vi "xyz-localisation.vi"(5 "Gy":dbl[][](array[numeric]), 7 "Gx":dbl[][](array[numeric]), 8 "R":dbl, 9 "weights":dbl[](array[numeric]), 10 "B points":dbl[][](array[numeric])=[[5.0, 3.0], [6.0, 6.0]], 11 "A points":dbl[][](array[numeric])=[[0.0, 1.0], [2.0, 3.0]]) -> (2 "dR":dbl[](array[numeric]), 3 "XYZ":dbl[](array[numeric]))   [LabVIEW 2015]
doc: "This vi calculates XYZ position of the particle. XY is found as a least square intersection point of gradient lines. Z position is a difference between sum of gradients to the left/bottom and rigth/up sides of particle center (requires calibration)\n\nINPUT\nR - radius of the window (should be >0.5)\nGx,Gy - horizontal and vertical local gradient images\nA points - 2xN array of first points that define lines\nB points - 2xN array of second points that define lines\nw - weights (1D array)\n\nOUTPUT\nXYZ - x,y position of the particle in pixels (for original image), z-value\ndR - distance from the center to each line (1D vector)\n\nAuthor: Anatolii Kashchuk"
panel:
  # "This vi finds centroid and z-value from the image of a particle\n\nAuthor: Anatolii Kashchuk"
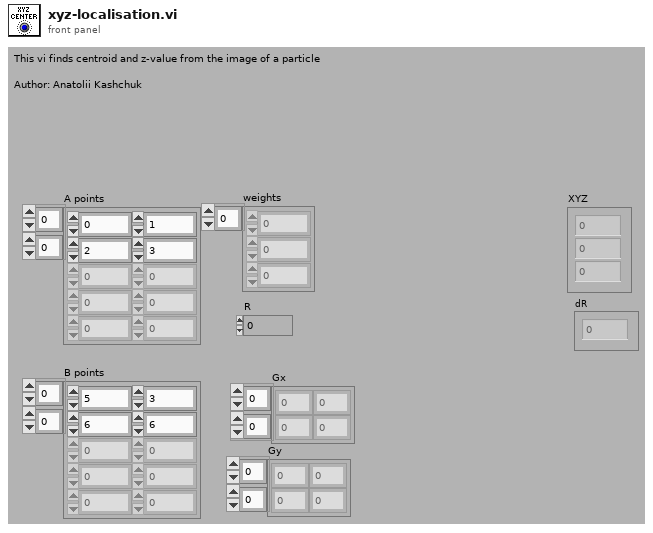
[diagram p1: front panel]
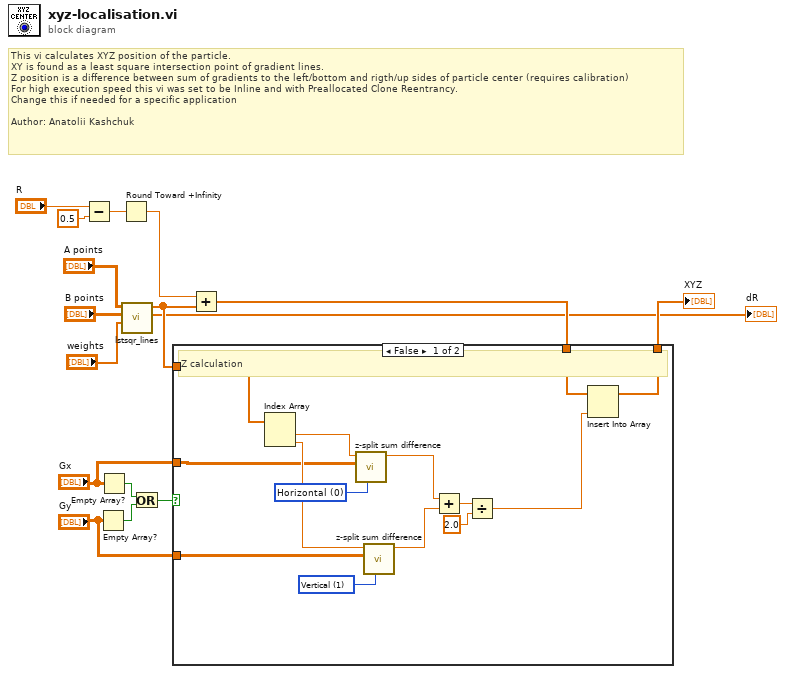
[diagram p0: block diagram]
diagram:
  # "This vi calculates XYZ position of the particle. \nXY is found as a least square intersection point of gradient lines. \nZ position is a difference between sum of gradients to the left/bottom and rigth/up sides of particle center (requires calibration)\nFor high execution speed this vi was set to be Inline and with Preallocated Clone Reentrancy. \nChange this if needed for a specific application\n\nAuthor: Anatolii Kashchuk"
  n1 = Subtract(x="R", y=0.5) -> (x-y=w11:dbl)
  n2 = Empty Array?(array="Gy") -> (empty?=w5:bool)
  n3 = Empty Array?(array="Gx") -> (empty?=w6:bool)
  n4 = Round Toward +Infinity(x=w11) -> (ceil(x): smallest int >= x=w12:dbl)
  n5 = call "lstsqr_lines.vi"("weights"="weights", "B points"="B points", "A points"="A points") -> ("dR"=→"dR":dbl[], "center"=w9:dbl[])  [unwired: 6 in, 1 out]
  n6 = Or(x=w6, y=w5) -> (x .or. y?=w4:bool)
  n7 = Add(x=w12, y=w9) -> (x+y=w8:dbl[])
  n8 = case shown="False" w4 {
    tunnel: w9 -> [w30 _]
    tunnel: w8 -> [w28 w31]
    tunnel: [w29 w31] -> w7
    tunnel: "Gx" -> [w22 _]
    tunnel: "Gy" -> [w26 _]
    frame False {
      w24 = u16 0 items=["Horizontal", "Vertical"] ("Text Ring")
      w27 = u16 1 items=["Horizontal", "Vertical"] ("Text Ring")
      # "Z calculation"
      n9 = Index Array(array=w30) -> (element #1=w23:dbl, element #2=w25:dbl)  [unwired: 2 in]
      n10 = call "z-split sum difference.vi"("split type"=w24, "G input"=w22, "center"=w23) -> ("difference"=w20:dbl)  [unwired: 6 in, 2 out]
      n11 = call "z-split sum difference.vi"("split type"=w27, "G input"=w26, "center"=w25) -> ("difference"=w21:dbl)  [unwired: 6 in, 2 out]
      n12 = Add(x=w20, y=w21) -> (x+y=w19:dbl)
      n13 = Divide(x=w19, y=2.0) -> (x/y=w17:dbl)
      n14 = Insert Into Array(array=w28, new element=w17) -> (w29:dbl[])  [unwired: 1 in]
    }
    frame True {
    }
  }
  "XYZ" <- w7
